vi "Get OS Information.vi"(11 "Steps to Reproduce":string) -> (3 "Metadata":string)   [LabVIEW 2014, in "Raspberry Pi Compatible Compiler for LabVIEW.lvlib"]
uses:
  Raspberry Pi Compatible Compiler for LabVIEW.lvlib
  Compile and Download App/Custom Controls/Local Setup Parameters.ctl
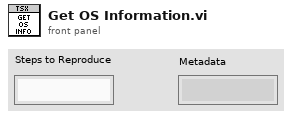
[diagram p1: front panel]
types:
  T1 = typedef "Raspberry Pi Compatible Compiler for LabVIEW.lvlib/Local Setup Parameters.ctl" = enum16{"Add Last VI", "Read Last VI", "Add Board IP", "Remove Board IP", "Read All Board IP", "Add Runtime Version", "Read Runtime Version", "Add Package Version", "Read Package Version", "Add VIPCheck Time", "Read VIPCheck Time"}
  T2 = enum32{"invalid app kind", "Development System", "Run Time System", "Student Edition", "Embedded LabVIEW", "Evaluation", "Custom"}
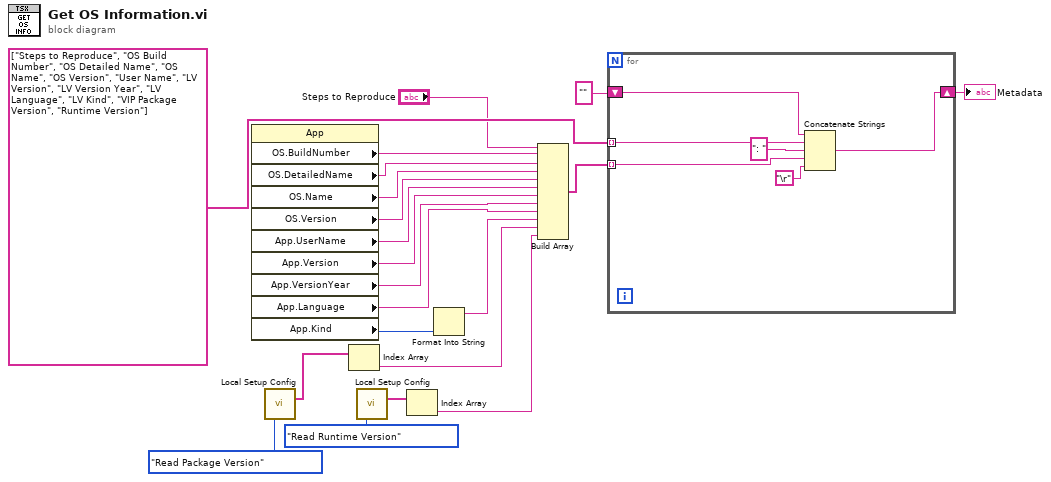
[diagram p0: block diagram]
diagram:
  n1 = property class="App"() -> ("OS.BuildNumber"=w21:string, "OS.DetailedName"=w20:string, "OS.Name"=w19:string, "OS.Version"=w18:string, "App.UserName"=w17:string, "App.Version"=w16:string, "App.VersionYear"=w15:string, "App.Language"=w14:string, "App.Kind"=w12:T2)  [unwired: 2 in, 2 out]
  n2 = call "Local Setup Config.vi"("Local Setup Param"=Local_Setup_Parameters."Read Package Version") -> ("KeyValues"=w5:string[])  [unwired: 11 in, 3 out]
  n3 = Index Array(array=w5) -> (element=w4:string)  [unwired: 1 in]
  n4 = call "Local Setup Config.vi"("Local Setup Param"=Local_Setup_Parameters."Read Runtime Version") -> ("KeyValues"=w2:string[])  [unwired: 11 in, 3 out]
  n5 = Index Array(array=w2) -> (element=w1:string)  [unwired: 1 in]
  n6 = Format Into String(w12) -> (resulting string=w11:string)  [unwired: 3 in, 1 out]
  n7 = Build Array("Steps to Reproduce", w21, w20, w19, w18, w17, w16, w15, w14, w11, w4, w1) -> (w13:string[])
  n8 = for {
    tunnel: w13 -> [w26] mode=indexing
    tunnel: string[] ["Steps to Reproduce", "OS Build Number", "OS Detailed Name", "OS Name", "OS Version", "User Name", "LV Version", "LV Version Year", "LV Language", "LV Kind", "VIP Package Version", "Runtime Version"] -> [w27] mode=indexing
    shift-right: [w23] -> w7
    shift-left: "" -> [w24]
    n9 = Concatenate Strings(w24, w27, ": " ("string"), w26, "\r") -> (w23:string)
  }
  "Metadata" <- w7
